vi "Handle Remove State Change.vi"(8 "error in (no error)":errorcluster, 10 "State":string, 11 "Routing Channel Ref in":T1 format="%.0x") -> (0 "error out":errorcluster, 2 "State to Display":string, 3 "Routing Channel Ref out":T1 format="%.0x")   [LabVIEW 2017, in "Routing and Faulting System Explorer.lvlib"]
uses:
  Routing and Faulting System Explorer.lvlib
  <vilib>/NI Veristand/Custom Device API/Custom Device Item Ref.ctl
  Scripting/Routing and Faulting Scripting.lvlib
  <vilib>/NI VeriStand/Custom Device API/Custom Device API.lvlib
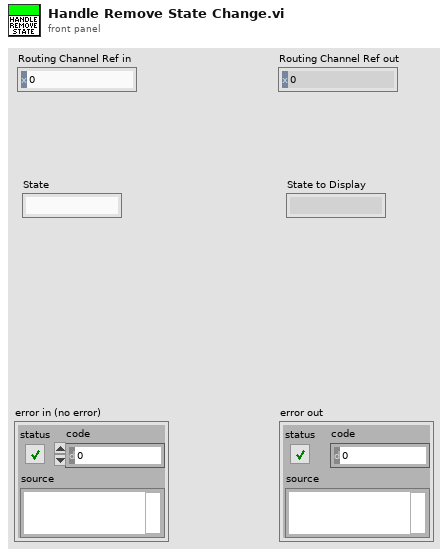
[diagram p1: front panel]
types:
  T1 = typedef "Custom Device API.lvlib/Custom Device Item Ref.ctl" = u64
  T2 = typedef "Routing and Faulting Shared.lvlib/Routing State.ctl" = cluster{"Name":string, "Description":string, "Value":i32, "Connection List":T3[]}
  T3 = typedef "Routing and Faulting Shared.lvlib/Connection.ctl" = cluster{"Resource":string, "Source":string, "Destination":string}
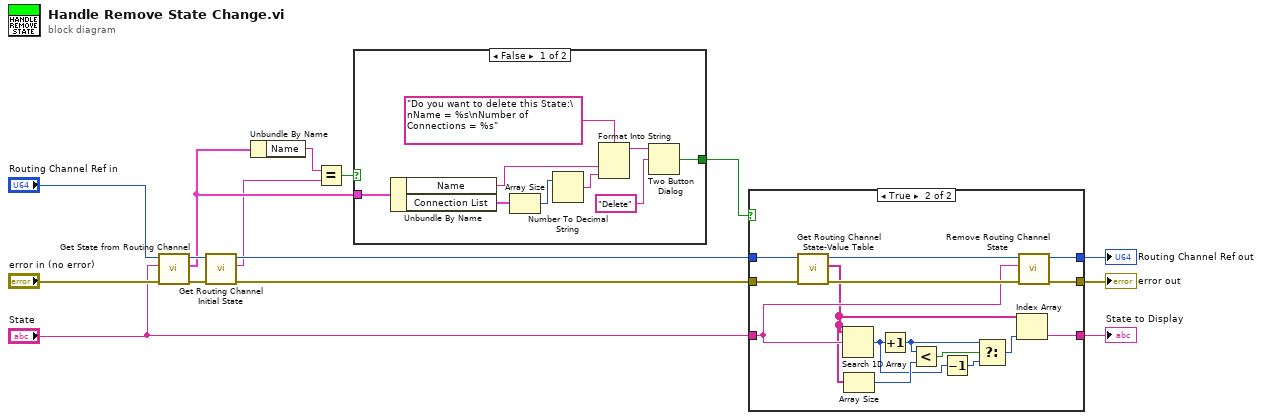
[diagram p0: block diagram]
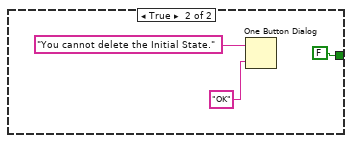
[diagram p2: hidden frame]
diagram:
  n1 = call "Get State from Routing Channel.vi"("error in (no error)"="error in (no error)", "State"="State", "Channel Ref in"="Routing Channel Ref in") -> ("error out"=w12:errorcluster, "State and Connections"=w4:T2, "Channel Ref out"=w6:T1)  [unwired: 6 in]
  n2 = call "Get Routing Channel Initial State.vi"("error in (no error)"=w12, "Channel Ref in"=w6) -> ("error out"=w7:errorcluster, "Initial State"=w3:string, "Channel Ref out"=w5:T1)  [unwired: 7 in]
  n3 = Unbundle By Name(w4) -> ("Name"=w2:string)
  n4 = Equal?(x=w2, y=w3) -> (x = y?=w1:bool)
  n5 = case shown="False" w1 {
    tunnel: w4 -> [w24 _]
    tunnel: [w16 FALSE ("T button?")] -> w10
    frame False {
      n6 = Unbundle By Name(w24) -> ("Name"=w22:string, "Connection List"=w21:T3[])
      n7 = Array Size(array=w21) -> (size(s)=w20:i32)
      n8 = Number To Decimal String(number=w20) -> (decimal integer string=w19:string)  [unwired: 1 in]
      n9 = Format Into String(format string="Do you want to delete this State:\nName = %s\nNumber of Connections = %s", w22, w19) -> (resulting string=w18:string)  [unwired: 2 in, 1 out]
      n10 = Two Button Dialog(message=w18, 2:"Delete" ("T button name (\"OK\")")) -> (T button?=w16:bool)  [unwired: 1 in]
    }
    frame True {
      n11 = One Button Dialog(message="You cannot delete the Initial State." ("format string"), button name ("OK")="OK" ("T button name (\"OK\")")) -> ()  [unwired: 1 out]
    }
  }
  n12 = case shown="True" w10 {
    tunnel: w5 -> [w29 w42]
    tunnel: "State" -> [w28 w39]
    tunnel: w7 -> [w30 w43]
    tunnel: [w30 w45] -> w11
    tunnel: [w29 w44] -> w9
    tunnel: [w28 w38] -> w8
    frame False {
    }
    frame True {
      n13 = call "Get Routing Channel State-Value Table.vi"("error in (no error)"=w43, "Channel Ref in"=w42) -> ("error out"=w40:errorcluster, "State Names"=w37:string[], "Channel Ref out"=w41:T1)  [unwired: 6 in, 1 out]
      n14 = Search 1D Array(1D array=w37, element=w39) -> (index of element=w33:i32)  [unwired: 1 in]
      n15 = Array Size(array=w37) -> (size(s)=w36:i32)
      n16 = Increment(x=w33) -> (x+1=w34:i32)
      n17 = Less?(x=w34, y=w36) -> (x < y?=w35:bool)
      n18 = Decrement(x=w33) -> (x-1=w32:i32)
      n19 = Select(t=w34, s=w35, f=w32) -> (s? t:f=w31:i32)
      n20 = Index Array(array=w37, index=w31) -> (element=w38:string)
      n21 = call "Remove Routing Channel State.vi"("error in (no error)"=w40, "State"=w39, "Channel Ref in"=w41) -> ("error out"=w45:errorcluster, "Channel Ref out"=w44:T1)  [unwired: 7 in]
    }
  }
  "error out" <- w11
  "Routing Channel Ref out" <- w9
  "State to Display" <- w8
